vi "CPUID.vi"() -> (3 "ToString":string)   [LabVIEW 2019]
uses:
  System.Management
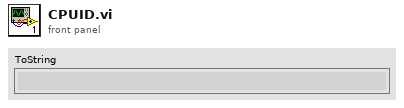
[diagram p1: front panel]
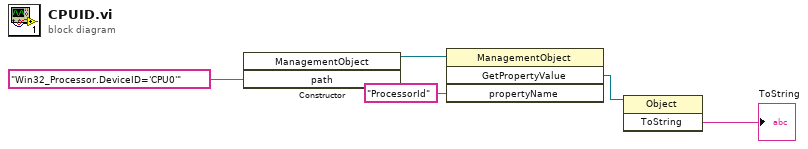
[diagram p0: block diagram]
diagram:
  n1 = constructor class="ManagementObject"("path"="Win32_Processor.DeviceID='CPU0'" ("queryString")) -> (reference out=w4:refnum<k24>)  [unwired: 3 in, 3 out]
  n2 = invoke class="ManagementObject" method="GetPropertyValue"(reference=w4, "propertyName"="ProcessorId") -> ("GetPropertyValue"=w2:refnum<k24>)  [unwired: 2 in, 3 out]
  n3 = invoke class="Object" method="ToString"(reference=w2) -> ("ToString"=→"ToString":string)  [unwired: 2 in, 2 out]
